vi "ExposeMessageCallback.vi"(4 "Callback Info":T1, 5 "Event Data":cluster{"sender":refnum<k24>, "e":refnum<k24>}, 6 "Control Ref":refnum<k24>, 7 "Event Common Data":T4) -> ()   [LabVIEW 2017]
uses:
  C:/Code/CMCryoSysCode/Expose/COM/CSCom/CSCom/bin/Release/CSCom.dll
  COM/CSCom/CSCom/bin/Release/CSCom.dll
  C:/Code/CMCryoSysCode/Expose/COM/CSCom/CSCom/bin/Release/WebsocketPipeCS.dll
  COM/CSCom/CSCom/bin/Release/WebsocketPipeCS.dll
  ExposeMessageCallbackInfo.ctl
  ExposeInfo.ctl
  ExposeHandlers.ctl
  ExposeMessage.ctl
  Events/ExposeMessageType.ctl
  Mapper/ExposeObjectMapNamepathData.ctl
  Mapper/ExposeMapperDataTypeEnum.ctl
  Mapper/ExposeObjectMapContainerTypeEnum.ctl
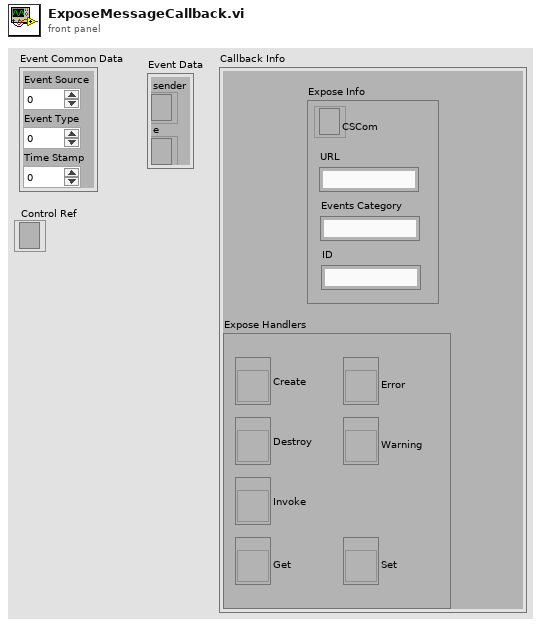
[diagram p1: front panel]
types:
  T1 = typedef "ExposeMessageCallbackInfo.ctl" = cluster{"Expose Info":T2, "Expose Handlers":T3}
  T2 = typedef "ExposeInfo.ctl" = cluster{"CSCom":refnum<k24>, "URL":string, "Events Category":string, "ID":string}
  T3 = typedef "ExposeHandlers.ctl" = cluster{"Create":refnum<vi>, "Destroy":refnum<vi>, "Invoke":refnum<vi>, "Get":refnum<vi>, "Set":refnum<vi>, "Error":refnum<vi>, "Warning":refnum<vi>}
  T4 = cluster{"Event Source":i32, "Event Type":u32, "Time Stamp":u32}
  T5 = typedef "ExposeMessage.ctl" = cluster{"Message Type":T6, "Text":string, "NamepathInfo":T7[]}
  T6 = typedef "ExposeMessageType.ctl" = i32
  T7 = typedef "ExposeObjectMapNamepathData.ctl" = cluster{"Type":T8, "Value":variant, "Namepath":string, "Container Type":T9}
  T8 = typedef "ExposeMapperDataTypeEnum.ctl" = enum16{"NotData", "int8", "byte", "int16", "uint16", "int32", "uint32", "int64", "uint64", "Single", "Double", "String", "Boolean", "Container"}
  T9 = typedef "ExposeObjectMapContainerTypeEnum.ctl" = enum16{"Value", "Array", "Waveform", "NetContainer"}
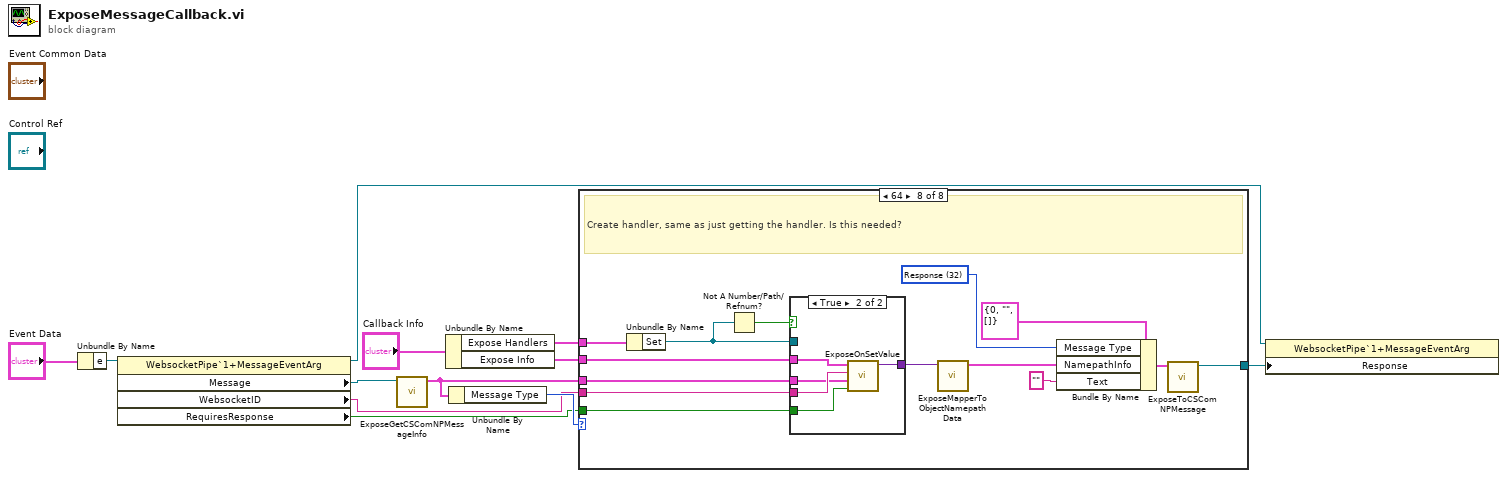
[diagram p0: block diagram]
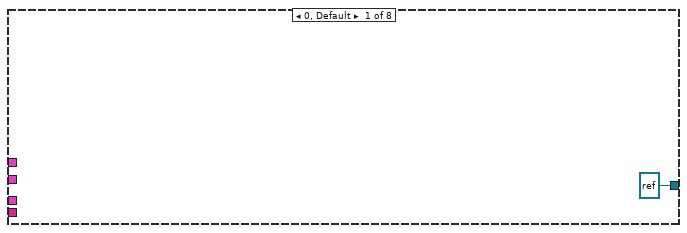
[diagram p2: hidden frame]
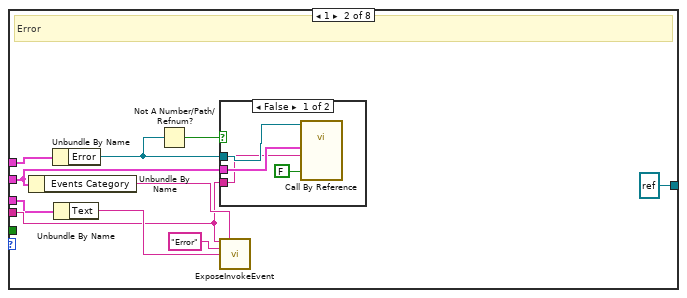
[diagram p3: hidden frame]
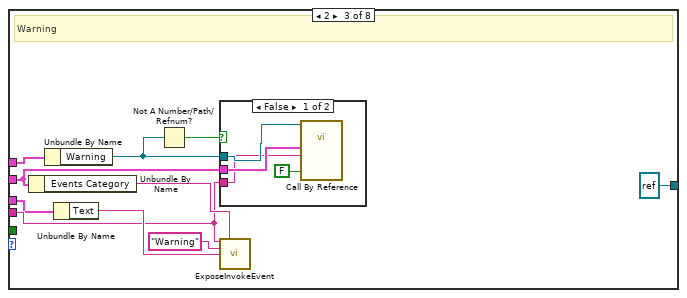
[diagram p5: hidden frame]
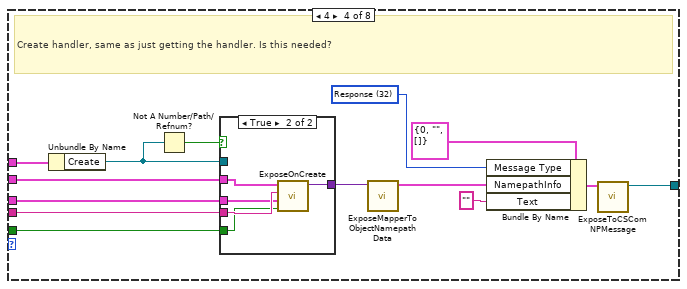
[diagram p7: hidden frame]
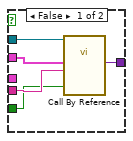
[diagram p8: hidden frame]
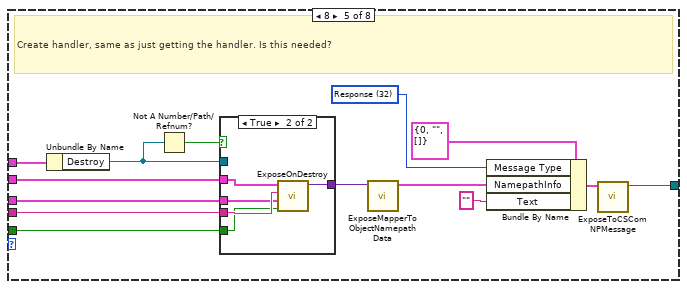
[diagram p9: hidden frame]
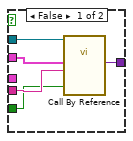
[diagram p10: hidden frame]
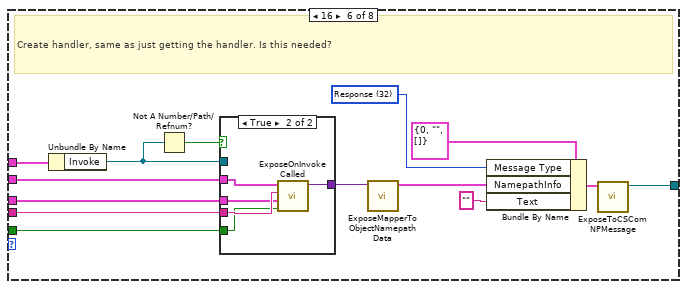
[diagram p11: hidden frame]
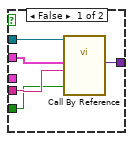
[diagram p12: hidden frame]
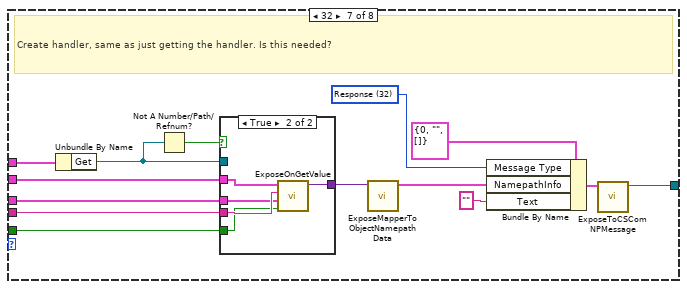
[diagram p13: hidden frame]
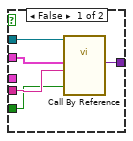
[diagram p14: hidden frame]
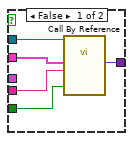
[diagram p15: hidden frame]
diagram:
  n1 = Unbundle By Name("Event Data") -> ("e"=w11:refnum<k24>)
  n2 = property class="WebsocketPipe`1+MessageEventArg"(reference=w11) -> (reference out=w5:refnum<k24>, "Message"=w10:refnum<k24>, "WebsocketID"=w8:string, "RequiresResponse"=w6:bool)  [unwired: 1 in, 1 out]
  n3 = call "ExposeGetCSComNPMessageInfo.vi"("NPMessage"=w10) -> ("MessageInfo"=w7:T5)  [unwired: 10 in]
  n4 = Unbundle By Name("Callback Info") -> ("Expose Handlers"=w1:T3, "Expose Info"=w2:T2)
  n5 = Unbundle By Name(w7) -> ("Message Type"=w9:T6)
  n6 = case shown="64" w9 {
    tunnel: w2 -> [_ w18 w32 w46 w70 w94 w118 w143]
    tunnel: w8 -> [_ w17 w31 w55 w79 w103 w127 w151]
    tunnel: w7 -> [_ w16 w30 w42 w66 w90 w114 w147]
    tunnel: w6 -> [_ _ _ w54 w78 w102 w126 w150]
    tunnel: [refnum<k24> refnum ("Response") refnum<k24> refnum ("Response") refnum<k24> refnum ("Response") w48 w72 w96 w120 w145] -> w4
    tunnel: w1 -> [_ w19 w33 w47 w71 w95 w119 w144]
    frame 0, Default {
    }
    frame 1 {
      # "Error"
      n7 = Unbundle By Name(w18) -> ("Events Category"=w22:string)
      n8 = Unbundle By Name(w19) -> ("Error"=w15:refnum<vi>)
      n9 = Unbundle By Name(w16) -> ("Text"=w21:string)
      n10 = Not A Number/Path/Refnum?(number/path/refnum=w15) -> (NaN/Path/Refnum?=w14:bool)
      n11 = case shown="False" w14 {
        tunnel: w15 -> [w27 _]
        tunnel: w18 -> [w26 _]
        tunnel: w17 -> [w25 _]
        frame False {
          n12 = call-by-ref "?"(reference=w27, "Requires Response"=FALSE, "HandlerID"=w25, "Expose Info"=w26) -> ()  [unwired: 9 in, 3 out]
        }
        frame True {
        }
      }
      n13 = call "ExposeInvokeEvent.vi"("ID"=w17, "Category"=w22, "name"="Error", "Data"=w21) -> ()  [unwired: 11 in, 1 out]
    }
    frame 2 {
      # "Warning"
      n14 = Unbundle By Name(w32) -> ("Events Category"=w36:string)
      n15 = Unbundle By Name(w33) -> ("Warning"=w28:refnum<vi>)
      n16 = Unbundle By Name(w30) -> ("Text"=w35:string)
      n17 = Not A Number/Path/Refnum?(number/path/refnum=w28) -> (NaN/Path/Refnum?=w29:bool)
      n18 = case shown="False" w29 {
        tunnel: w28 -> [w41 _]
        tunnel: w32 -> [w40 _]
        tunnel: w31 -> [w39 _]
        frame False {
          n19 = call-by-ref "?"(reference=w41, "Requires Response"=FALSE, "HandlerID"=w39, "Expose Info"=w40) -> ()  [unwired: 9 in, 3 out]
        }
        frame True {
        }
      }
      n20 = call "ExposeInvokeEvent.vi"("ID"=w31, "Category"=w36, "name"="Warning", "Data"=w35) -> ()  [unwired: 11 in, 1 out]
    }
    frame 4 {
      w51 = T6 32 items=["Error"=1, "Warning"=2, "Create"=4, "Destroy"=8, "Invoke"=16, "Response"=32] ("Message Type")
      # "Create handler, same as just getting the handler. Is this needed?"
      n21 = Unbundle By Name(w47) -> ("Create"=w44:refnum<vi>)
      n22 = Not A Number/Path/Refnum?(number/path/refnum=w44) -> (NaN/Path/Refnum?=w43:bool)
      n23 = case shown="True" w43 {
        tunnel: w44 -> [w60 _]
        tunnel: w55 -> [w59 w64]
        tunnel: w54 -> [w58 w62]
        tunnel: [w57 w61] -> w53
        tunnel: w46 -> [w56 w65]
        tunnel: w42 -> [_ w63]
        frame False {
          n24 = call-by-ref "?"(reference=w60, "Requires Response"=w58, "HandlerID"=w59, "Expose Info"=w56) -> ("Response"=w57:variant)  [unwired: 9 in, 2 out]
        }
        frame True {
          n25 = call "ExposeOnCreate.vi"("Requires Response"=w62, "Message"=w63, "HandlerID"=w64, "Expose Info"=w65) -> ("Response"=w61:variant)  [unwired: 7 in]
        }
      }
      n26 = call "ExposeMapperToObjectNamepathData.vi"("Value"=w53) -> ("Object map"=w45:T7[])  [unwired: 10 in]
      n27 = Bundle By Name(cluster=T5 {"Message Type"=0, "Text"="", "NamepathInfo"=[]} ("ExposeMessage"), "Message Type"=w51, "NamepathInfo"=w45, "Text"="") -> (w49:T5)
      n28 = call "ExposeToCSComNPMessage.vi"("Message"=w49) -> (".NET Refnum out"=w48:refnum<k24>)  [unwired: 10 in]
    }
    frame 8 {
      w75 = T6 32 items=["Error"=1, "Warning"=2, "Create"=4, "Destroy"=8, "Invoke"=16, "Response"=32] ("Message Type")
      # "Create handler, same as just getting the handler. Is this needed?"
      n29 = Unbundle By Name(w71) -> ("Destroy"=w67:refnum<vi>)
      n30 = Not A Number/Path/Refnum?(number/path/refnum=w67) -> (NaN/Path/Refnum?=w68:bool)
      n31 = case shown="True" w68 {
        tunnel: w67 -> [w84 _]
        tunnel: w79 -> [w83 w88]
        tunnel: w78 -> [w82 w86]
        tunnel: [w81 w85] -> w77
        tunnel: w70 -> [w80 w89]
        tunnel: w66 -> [_ w87]
        frame False {
          n32 = call-by-ref "?"(reference=w84, "Requires Response"=w82, "HandlerID"=w83, "Expose Info"=w80) -> ("Response"=w81:variant)  [unwired: 9 in, 2 out]
        }
        frame True {
          n33 = call "ExposeOnDestroy.vi"("Requires Response"=w86, "Message"=w87, "HandlerID"=w88, "Expose Info"=w89) -> ("Response"=w85:variant)  [unwired: 7 in]
        }
      }
      n34 = call "ExposeMapperToObjectNamepathData.vi"("Value"=w77) -> ("Object map"=w69:T7[])  [unwired: 10 in]
      n35 = Bundle By Name(cluster=T5 {"Message Type"=0, "Text"="", "NamepathInfo"=[]} ("ExposeMessage"), "Message Type"=w75, "NamepathInfo"=w69, "Text"="") -> (w73:T5)
      n36 = call "ExposeToCSComNPMessage.vi"("Message"=w73) -> (".NET Refnum out"=w72:refnum<k24>)  [unwired: 10 in]
    }
    frame 16 {
      w99 = T6 32 items=["Error"=1, "Warning"=2, "Create"=4, "Destroy"=8, "Invoke"=16, "Response"=32] ("Message Type")
      # "Create handler, same as just getting the handler. Is this needed?"
      n37 = Unbundle By Name(w95) -> ("Invoke"=w92:refnum<vi>)
      n38 = Not A Number/Path/Refnum?(number/path/refnum=w92) -> (NaN/Path/Refnum?=w91:bool)
      n39 = case shown="True" w91 {
        tunnel: w92 -> [w108 _]
        tunnel: w103 -> [w107 w112]
        tunnel: w102 -> [w106 w110]
        tunnel: [w105 w109] -> w101
        tunnel: w94 -> [w104 w113]
        tunnel: w90 -> [_ w111]
        frame False {
          n40 = call-by-ref "?"(reference=w108, "Requires Response"=w106, "HandlerID"=w107, "Expose Info"=w104) -> ("Response"=w105:variant)  [unwired: 9 in, 2 out]
        }
        frame True {
          n41 = call "ExposeOnInvokeCalled.vi"("Requires Response"=w110, "Message"=w111, "HandlerID"=w112, "Expose Info"=w113) -> ("Response"=w109:variant)  [unwired: 7 in]
        }
      }
      n42 = call "ExposeMapperToObjectNamepathData.vi"("Value"=w101) -> ("Object map"=w93:T7[])  [unwired: 10 in]
      n43 = Bundle By Name(cluster=T5 {"Message Type"=0, "Text"="", "NamepathInfo"=[]} ("ExposeMessage"), "Message Type"=w99, "NamepathInfo"=w93, "Text"="") -> (w97:T5)
      n44 = call "ExposeToCSComNPMessage.vi"("Message"=w97) -> (".NET Refnum out"=w96:refnum<k24>)  [unwired: 10 in]
    }
    frame 32 {
      w123 = T6 32 items=["Error"=1, "Warning"=2, "Create"=4, "Destroy"=8, "Invoke"=16, "Response"=32] ("Message Type")
      # "Create handler, same as just getting the handler. Is this needed?"
      n45 = Unbundle By Name(w119) -> ("Get"=w116:refnum<vi>)
      n46 = Not A Number/Path/Refnum?(number/path/refnum=w116) -> (NaN/Path/Refnum?=w115:bool)
      n47 = case shown="True" w115 {
        tunnel: w116 -> [w132 _]
        tunnel: w127 -> [w131 w136]
        tunnel: w126 -> [w130 w135]
        tunnel: [w129 w133] -> w125
        tunnel: w118 -> [w128 w137]
        tunnel: w114 -> [_ w134]
        frame False {
          n48 = call-by-ref "?"(reference=w132, "Requires Response"=w130, "HandlerID"=w131, "Expose Info"=w128) -> ("Response"=w129:variant)  [unwired: 9 in, 2 out]
        }
        frame True {
          n49 = call "ExposeOnGetValue.vi"("Requires Response"=w135, "Message"=w134, "HandlerID"=w136, "Expose Info"=w137) -> ("Response"=w133:variant)  [unwired: 7 in]
        }
      }
      n50 = call "ExposeMapperToObjectNamepathData.vi"("Value"=w125) -> ("Object map"=w117:T7[])  [unwired: 10 in]
      n51 = Bundle By Name(cluster=T5 {"Message Type"=0, "Text"="", "NamepathInfo"=[]} ("ExposeMessage"), "Message Type"=w123, "NamepathInfo"=w117, "Text"="") -> (w121:T5)
      n52 = call "ExposeToCSComNPMessage.vi"("Message"=w121) -> (".NET Refnum out"=w120:refnum<k24>)  [unwired: 10 in]
    }
    frame 64 {
      w148 = T6 32 items=["Error"=1, "Warning"=2, "Create"=4, "Destroy"=8, "Invoke"=16, "Response"=32] ("Message Type")
      # "Create handler, same as just getting the handler. Is this needed?"
      n53 = Unbundle By Name(w144) -> ("Set"=w142:refnum<vi>)
      n54 = Not A Number/Path/Refnum?(number/path/refnum=w142) -> (NaN/Path/Refnum?=w141:bool)
      n55 = case shown="True" w141 {
        tunnel: w151 -> [w156 w160]
        tunnel: w150 -> [w155 w158]
        tunnel: [w154 w157] -> w149
        tunnel: w147 -> [_ w159]
        tunnel: w143 -> [w153 w161]
        tunnel: w142 -> [w152 _]
        frame False {
          n56 = call-by-ref "?"(reference=w152, "Requires Response"=w155, "HandlerID"=w156, "Expose Info"=w153) -> ("Response"=w154:variant)  [unwired: 9 in, 2 out]
        }
        frame True {
          n57 = call "ExposeOnSetValue.vi"("Requires Response"=w158, "Message"=w159, "HandlerID"=w160, "Expose Info"=w161) -> ("Response"=w157:variant)  [unwired: 7 in]
        }
      }
      n58 = call "ExposeMapperToObjectNamepathData.vi"("Value"=w149) -> ("Object map"=w138:T7[])  [unwired: 10 in]
      n59 = Bundle By Name(cluster=T5 {"Message Type"=0, "Text"="", "NamepathInfo"=[]} ("MessageInfo"), "Message Type"=w148, "NamepathInfo"=w138, "Text"="") -> (w139:T5)
      n60 = call "ExposeToCSComNPMessage.vi"("Message"=w139) -> (".NET Refnum out"=w145:refnum<k24>)  [unwired: 10 in]
    }
  }
  n61 = property class="WebsocketPipe`1+MessageEventArg"(reference=w5, "Response"=w4) -> ()  [unwired: 1 in, 2 out]
